vi "GetAlazar_PassData.vi"(0 "AlazarCluster":T5, 1 "Digitizer Settings":T1={"Digitizer delay (us) "=0.0, "rf points per line"=2048, "lines per plane"=128, "Samp Rate (Hz)"=100000000.0, "Additional dig delay (us)"=0.0, "Voltage Scale"=0.4, "Pre-Looks"=0, "Offset delay (us)"=0.0, "bits A/D"=8, "Avg Num"=1, "DigTimeOut"=5.0, "Rel Dig Delay"=0.0, "Dig Ch"=0, "LeCroyCluster"={"LeCroy Channels"=[TRUE, FALSE, FALSE, FALSE], "LC read pt offset"=0.0, "Sweep Avg"=FALSE}, "Main Digitizer"=enum."NI Digitizer", "Dig Config"=enum."Single channel", "Digitizer ID Cluster"={"Acqiris/Alazar/SP ID"=[], "NI Instr Handles"=[], "LeCroy VISA"="", "GaGe Handle"={"Handle"=0, "Sample size"=0, "Resolution"=0, "Offset"=0, "Channels"=0, "Boards"=0}, "ATS Ref"="ATS9350", "Acqiris Address"=["PCI::INSTR0"], "ADQRef"=refnum, "adq_cu_ptr"=refnum}, "Trigger Settings"={"Trig Source"=1, "Trig Coupling"=0, "Trig Slope"=0, "Level (mV)"=1500.0}, "Bulk Acq"=FALSE, "Bulk Start Indexes"=[], "Data Ref RF"=refnum, "NI ID/Channel"=[], "Total Dig CH"=1, "Xtra Ann Trig delay (us)"=10.0, "Fix Z Delay?"=FALSE, "One Way Transmission?"=FALSE, "Data Ref Log"=refnum} {"Trigger Settings"."Trig Slope" items=["Positive", "Negative"]; "Trigger Settings"."Level (mV)" format="%.2f"; "Trigger Settings"."Trig Coupling" items=["DC 1 MOhm", "AC 1 MOhm", "DC 50 Ohm", "AC 50 Ohm"]; "Trigger Settings"."Trig Source" items=["Chan 1", "External"]; "Rel Dig Delay" format="%.2f"; "DigTimeOut" format="%.2f"; "Avg Num" min=1; "Offset delay (us)" format="%.2f"; "Additional dig delay (us)" format="%.2f"; "Digitizer delay (us)" format="%.2f"}, 7 "errorin":errorcluster, 8 "File Array":string[](array[string]), 10 "lines per plane":i32, 15 "Reverse?":bool) -> (17 "Raw VGain (scale)":dbl, 18 "Gain Array":T7(array[cluster]), 20 "Array out":i16[][][](array[numeric]), 21 "VGain (dB)":dbl, 27 "error out":errorcluster)   [LabVIEW 2022 SP3]
uses:
  -ScanSystem/DataHandling/ReverseData.vi
  -DigitizerRoutines/DigitizerSettings.ctl
  -DigitizerRoutines/DigitizerID.ctl
  -DigitizerRoutines/Digitizer.ctl
  -DigitizerRoutines/DigConfig.ctl
  C:/Windows/System32/ADQAPI_dotNet_helper.dll
panel:
  out "Voltage Scale":T6
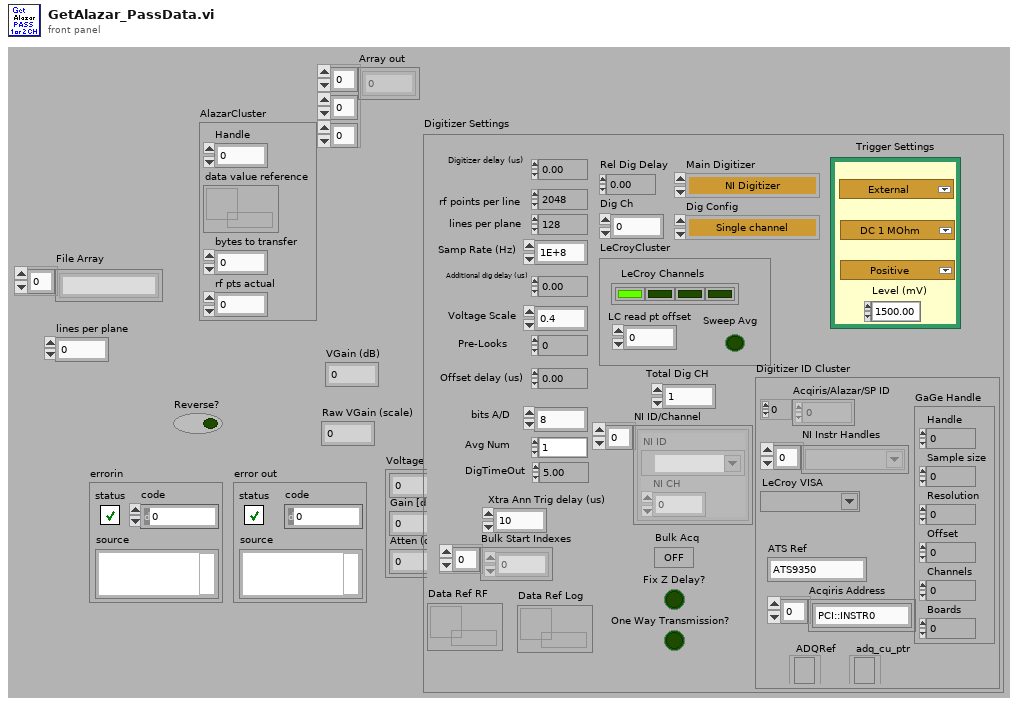
[diagram p1: front panel]
types:
  T1 = typedef "DigitizerSettings.ctl" = cluster{"Digitizer delay (us) ":dbl, "rf points per line":i32, "lines per plane":i32, "Samp Rate (Hz)":dbl, "Additional dig delay (us)":dbl, "Voltage Scale":dbl, "Pre-Looks":i32, "Offset delay (us)":dbl, "bits A/D":i8, "Avg Num":i32, "DigTimeOut":sgl, "Rel Dig Delay":sgl, "Dig Ch":i32, "LeCroyCluster":cluster{"LeCroy Channels":bool[], "LC read pt offset":dbl, "Sweep Avg":bool}, "Main Digitizer":T2, "Dig Config":T3, "Digitizer ID Cluster":T4, "Trigger Settings":cluster{"Trig Source":u16, "Trig Coupling":u16, "Trig Slope":u16, "Level (mV)":dbl}, "Bulk Acq":bool, "Bulk Start Indexes":i32[], "Data Ref RF":refnum<data-value>, "NI ID/Channel":cluster{"NI ID":refnum<k15>, "NI CH":i32}[], "Total Dig CH":i32, "Xtra Ann Trig delay (us)":dbl, "Fix Z Delay?":bool, "One Way Transmission?":bool, "Data Ref Log":refnum<data-value>}
  T2 = typedef "Digitizer.ctl" = enum16{"Acqiris Digitizer", "NI Digitizer", "LeCroy", "GaGe", "AlazarTech", "No Digitizer", "Teledyne"}
  T3 = typedef "DigConfig.ctl" = enum16{"Single channel", "2 Chans w/ 2 Acqiris", "2 Chans w/ 1 Acqiris", "5-CH Pulser New", "5-CH pulser w/ ann array", "5-pass style ann array", "Empty"}
  T4 = typedef "DigitizerID.ctl" = cluster{"Acqiris/Alazar/SP ID":u32[], "NI Instr Handles":refnum<k15>[], "LeCroy VISA":refnum<visa-resource-name>, "GaGe Handle":cluster{"Handle":u32, "Sample size":u32, "Resolution":i32, "Offset":i32, "Channels":u32, "Boards":u32}, "ATS Ref":string, "Acqiris Address":string[], "ADQRef":refnum<k24>, "adq_cu_ptr":refnum<k24>}
  T5 = cluster{"Handle":u32, "data value reference":refnum<data-value>, "bytes to transfer":u32, "rf pts actual":u32}
  T6 = cluster{sgl, "Gain [dB]  ":sgl, "Atten (dB)":sgl}
  T7 = cluster{sgl, "Gain [dB]  ":sgl, "Atten (dB)":sgl}[]
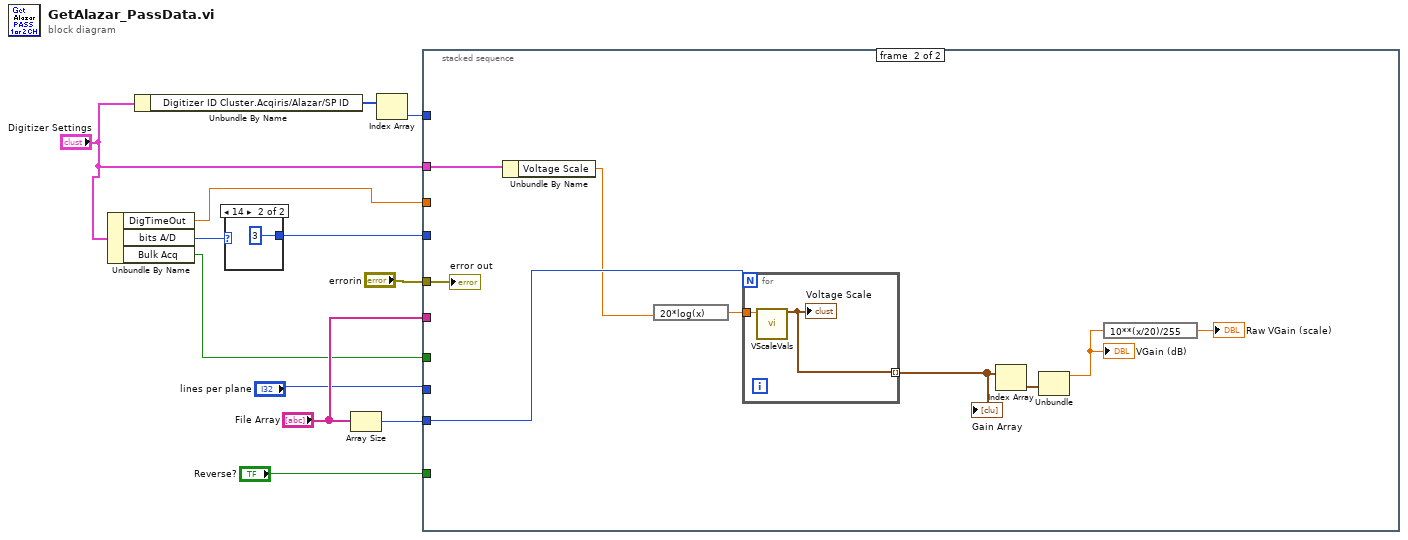
[diagram p0: block diagram]
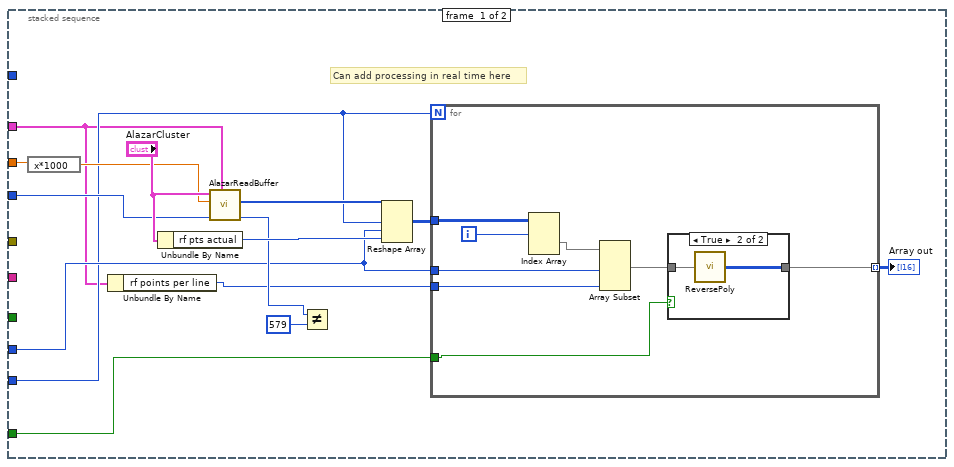
[diagram p3: hidden frame]
diagram:
  n1 = Unbundle By Name("Digitizer Settings") -> ("DigTimeOut"=w3:sgl, "bits A/D"=w4:i8, "Bulk Acq"=w1:bool)
  n2 = Unbundle By Name("Digitizer Settings") -> ("Digitizer ID Cluster.Acqiris/Alazar/SP ID"=w7:u32[])
  n3 = case shown="14" w4 {
    tunnel: [_ u16 3 ("Extra Shift")] -> w5
    frame 0, Default {
    }
    frame 14 {
    }
  }
  n4 = Array Size(array="File Array") -> (size(s)=w12:i32)
  n5 = Index Array(array=w7) -> (element=w6:u32)  [unwired: 1 in]
  n6 = stacked-sequence {
    tunnel: w3 -> [w20 _]
    tunnel: "lines per plane" -> [w22 _]
    tunnel: "File Array" -> [_ _]
    tunnel: "Reverse?" -> [w21 _]
    tunnel: "errorin" -> [_ w46]
    tunnel: w12 -> [w17 w47]
    tunnel: w1 -> [_ _]
    tunnel: w6 -> [_ _]
    tunnel: w5 -> [w18 _]
    tunnel: "Digitizer Settings" -> [w15 w41]
    frame #0 {
      # "Can add processing in real time here"
      n7 = expression code="x*1000"(w20) -> (w19:sgl)
      n8 = Unbundle By Name(w15) -> ("rf points per line"=w14:i32)
      n9 = Unbundle By Name("AlazarCluster") -> ("rf pts actual"=w26:u32)
      n10 = call "AlazarReadBuffer.vi"("Digitizer Settings"=w15, "Extra Shift"=w18, "time out"=w19, "AlazarCluster"="AlazarCluster") -> ("Return Code"=w25:u32, "Data Array"=w27:i16[])  [unwired: 5 in, 1 out]
      n11 = Not Equal?(x=w25, y=u32 579) -> ()  [unwired: 1 out]
      n12 = Reshape Array(w27, w17, w22, w26) -> (w28:i16[][][])
      n13 = for {
        N: w17 -> [_]
        tunnel: w28 -> [w36]
        tunnel: w14 -> [w35]
        tunnel: w22 -> [w34]
        tunnel: w21 -> [w33]
        tunnel: [w29] -> w16 mode=indexing
        i -> [w30]
        n14 = Index Array(array=w36, index (dim 0)=w30) -> (element=w31:i16[][])  [unwired: 2 in]
        n15 = Array Subset(array=w31, length (row)=w34, length (col)=w35) -> (w32:i16[][])  [unwired: 2 in]
        n16 = case shown="True" w33 {
          tunnel: [w37 w39] -> w29
          tunnel: w32 -> [w37 w38]
          frame False {
          }
          frame True {
            n17 = call-poly "ReversePoly.vi"("Array in"=w38) -> ("Array out"=w39:i16[][])
          }
        }
      }
      "Array out" <- w16
    }
    frame #1 {
      n18 = Unbundle By Name(w41) -> ("Voltage Scale"=w40:dbl)
      n19 = expression code="20*log(x)"(w40) -> (w48:dbl)
      n20 = for {
        N: w47 -> [_]
        tunnel: [w49] -> w42 mode=indexing
        tunnel: w48 -> [w50]
        n21 = call "VScaleVals.vi"("Full Scale"=w50) -> ("Voltage Scale"=w49:T6)  [unwired: 8 in, 2 out]
        "Voltage Scale" <- w49
      }
      "Gain Array" <- w42
      n22 = Index Array(array=w42) -> (element=w45:T6)  [unwired: 1 in]
      n23 = Unbundle(w45) -> (w44:sgl)  [unwired: 2 out]
      "VGain (dB)" <- w44
      n24 = expression code="10**(x/20)/255"(w44) -> (→"Raw VGain (scale)":sgl)
      "error out" <- w46
    }
  }
